vi "仿真信号.vi"() -> ()   [LabVIEW 2018]
panel:
  in  "Seed Number":dbl=-1.0 caption="种子值"
  in  "Offset":dbl caption="偏移量"
  in  "Phase":dbl caption="相位"
  in  "Amplitude":dbl=1.0 caption="幅值"
  in  "Frequency":dbl=10.1 caption="频率"
  in  "停止":bool
  out "波形图":dynamicdata(graph)
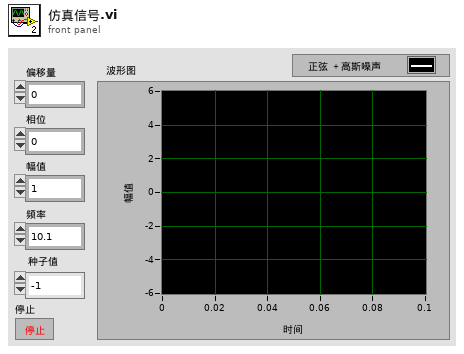
[diagram p1: front panel]
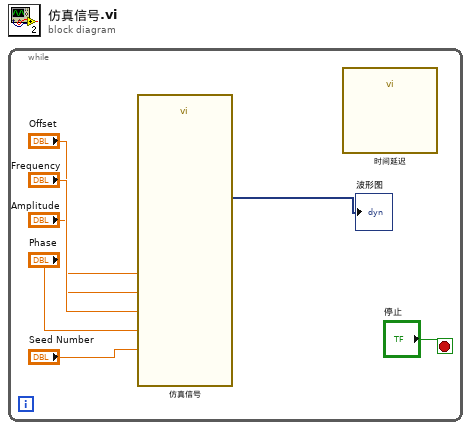
[diagram p0: block diagram]
diagram:
  n1 = while {
    stop <- "停止" stop-if-true
    n2 = call "仿真信号"("Offset"="Offset", "Frequency"="Frequency", "Amplitude"="Amplitude", "Phase"="Phase", "Seed Number"="Seed Number") -> ("正弦与高斯噪声"=→"波形图":dynamicdata)  [unwired: 9 in, 1 out]
    n3 = call "时间延迟"() -> ()  [unwired: 11 in, 1 out]
  }
